vi "Manual Enabled.vi"(8 "error in":errorcluster, 11 "Base Software in":refnum<class "Base Software.lvclass">) -> (0 "error out":errorcluster, 1 "Warning Message":string, 2 "Enabled?":bool, 3 "Base Software out":refnum<class "Base Software.lvclass">)   [LabVIEW 2019, in "Base Software.lvlib" / "Main.lvlib" / "Base Software.lvclass"]
uses:
  Project/Base Software.lvclass
  Project/Base Software.lvclass/Base Software.ctl
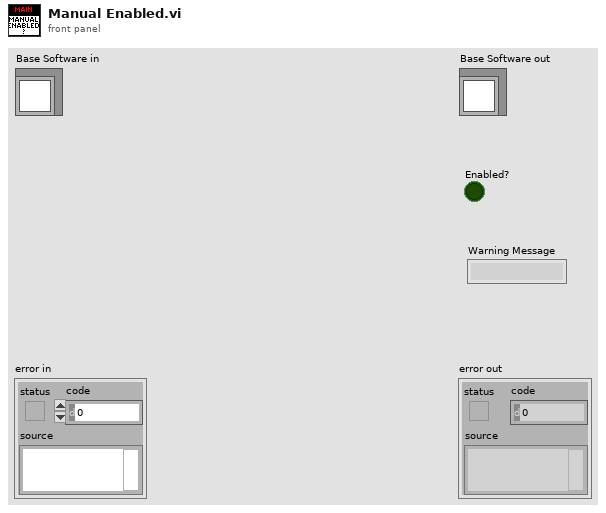
[diagram p1: front panel]
types:
  T1 = enum8{"Enabled", "Disabled", "Disabled and Grayed Out"}
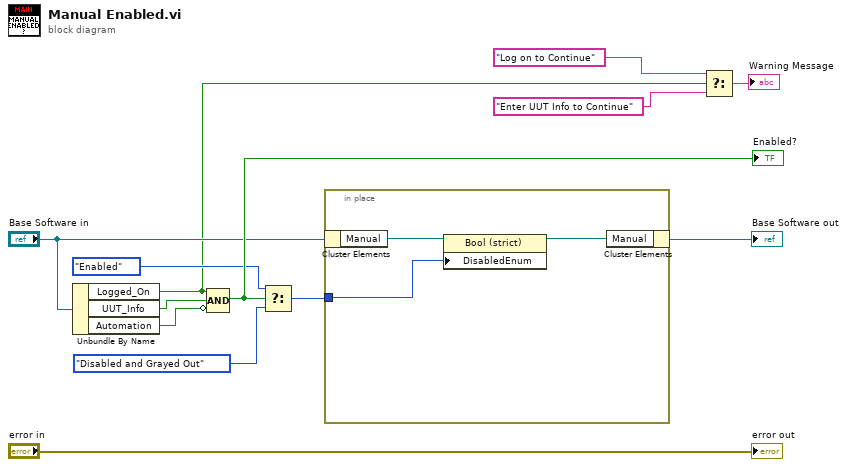
[diagram p0: block diagram]
diagram:
  n1 = Unbundle By Name("Base Software in") -> ("Logged_On"=w4:bool, "UUT_Info"=w12:bool, "Automation"=w11:bool)
  n2 = Compound Arithmetic op=AND(w4, w12, invert w11) -> (w10:bool)
  "Enabled?" <- w10
  n3 = Select(t=T1."Enabled" ("Disabled"), s=w10, f=T1."Disabled and Grayed Out" ("Disabled")) -> (s? t:f=w5:T1)
  n4 = in-place {
    in-place-border: w5 -> [w16]
    n5 = in-place-cluster #1("Base Software in") -> ("Manual"=w15:refnum<vi>)
    n6 = property class="Bool (strict)"(reference=w15, "DisabledEnum"=w16) -> (reference out=w14:refnum<vi>)  [unwired: 1 in, 1 out]
    n7 = in-place-cluster #1("Manual"=w14) -> (→"Base Software out":refnum<class "Base Software.lvclass">)
  }
  n8 = Select(t="Log on to Continue", s=w4, f="Enter UUT Info to Continue") -> (s? t:f=→"Warning Message":string)
  "error out" <- "error in"
